vi "Reset.vi"(8 "error in (no error)":errorcluster, 11 "VISA resource name":refnum<visa-resource-name>) -> (0 "error out":errorcluster, 3 "VISA resource name out":refnum<visa-resource-name>)   [LabVIEW 2019, in "Keithley 6517.lvlib"]
doc: "Resets the instrument and then sends a set of default setup commands to the instrument."
uses:
  Keithley 6517.lvlib
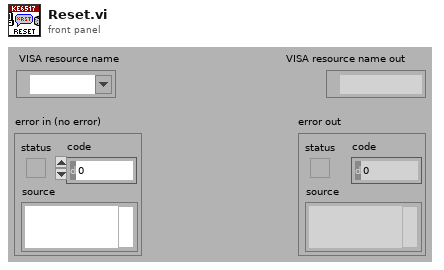
[diagram p1: front panel]
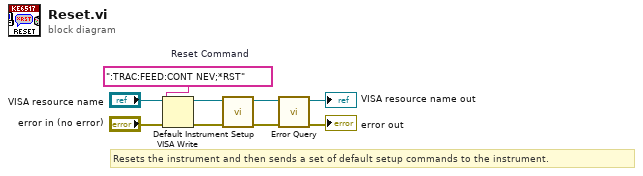
[diagram p0: block diagram]
diagram:
  w7 = ":TRAC:FEED:CONT NEV;*RST"  # Reset Command
  # "Resets the instrument and then sends a set of default setup commands to the instrument."
  n1 = VISA Write(VISA resource name="VISA resource name", write buffer=w7, error in (no error)="error in (no error)") -> (VISA resource name out=w5:refnum<visa-resource-name>, error out=w6:errorcluster)  [unwired: 1 out]
  n2 = call "Default Instrument Setup.vi"("error in (no error)"=w6, "VISA resource name"=w5) -> ("error out"=w4:errorcluster, "VISA resource name out"=w3:refnum<visa-resource-name>)  [unwired: 8 in]
  n3 = call "Error Query.vi"("error in (no error)"=w4, "VISA resource name"=w3) -> ("error out"=→"error out":errorcluster, "VISA resource name out"=→"VISA resource name out":refnum<visa-resource-name>)  [unwired: 6 in, 2 out]
